vi "Play.vi"(0 "Refnum in":refnum<k20>, 1 "Track Enable":T1={"Track_0 _Enable "=TRUE, "Track_1 _Enable "=TRUE, "Track_2 _Enable "=TRUE, "Track_3 _Enable "=TRUE}, 5 "Track (File) References":T2, 7 "Sample Index":i32, 9 "Sample Block Size":i32, 11 "error in (no error)":errorcluster) -> (4 "Refnum out":refnum<k20>, 6 "Track (File) References Out":T2, 15 "error out":errorcluster)   [LabVIEW 2014]
uses:
  Controls/Track (File) References.ctl
  Controls/Track Enable.ctl
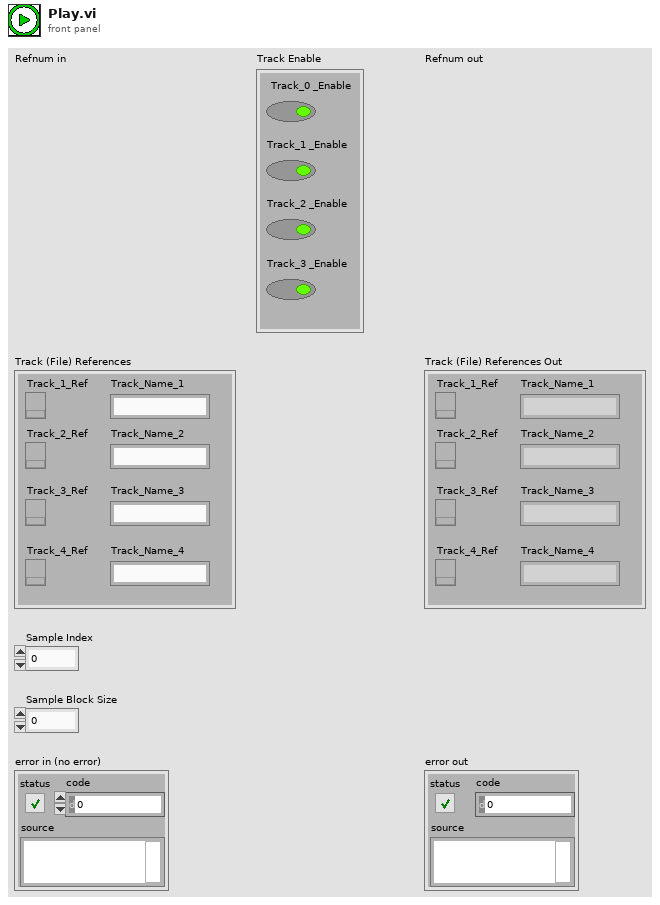
[diagram p1: front panel]
types:
  T1 = typedef "Track Enable.ctl" = cluster{"Track_0 _Enable ":bool, "Track_1 _Enable ":bool, "Track_2 _Enable ":bool, "Track_3 _Enable ":bool}
  T2 = typedef "Track (File) References.ctl" = cluster{"Track_1_Ref":refnum<k34>, "Track_2_Ref":refnum<k34>, "Track_3_Ref":refnum<k34>, "Track_4_Ref":refnum<k34>, "Track_Name_1":string, "Track_Name_2":string, "Track_Name_3":string, "Track_Name_4":string}
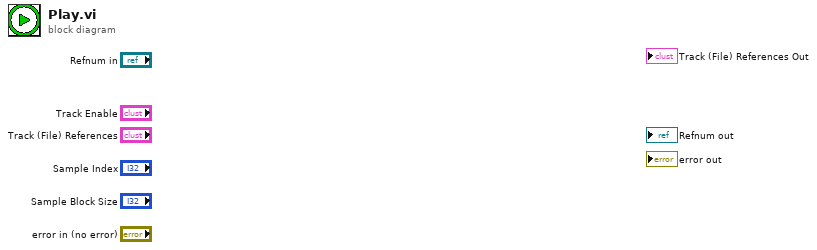
[diagram p0: block diagram]
diagram:
